vi "Read wires.vi"(8 "error in (no error)":errorcluster, 11 "BlockDiagram in":refnum<class "BlockDiagram.lvclass">) -> (0 "error out":errorcluster, 2 "wires":refnum<class "Wire.lvclass">[](array[class]), 3 "BlockDiagram out":refnum<class "BlockDiagram.lvclass">)   [LabVIEW 2023, in "TLC_Scripto.lvlib" / "BlockDiagram.lvclass"]
uses:
  BlockDiagram.lvclass
  Wire/Wire.lvclass
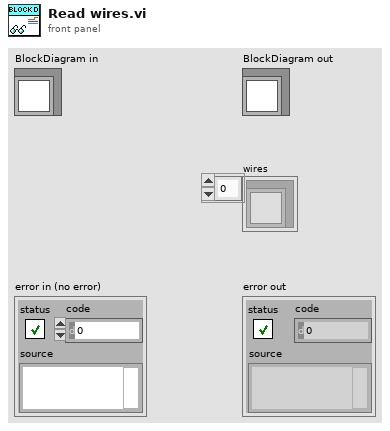
[diagram p1: front panel]
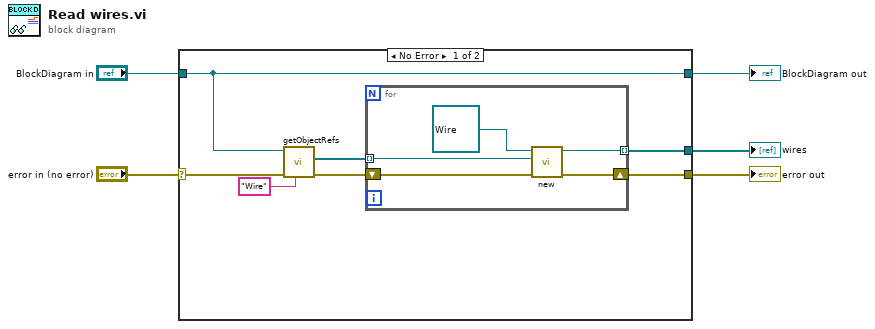
[diagram p0: block diagram]
diagram:
  n1 = case shown="No Error" "error in (no error)" {
    selector: "error in (no error)" -> [w10 w19]
    tunnel: [w7 w19] -> w4
    tunnel: [w12 w18] -> w2
    tunnel: "BlockDiagram in" -> [w12 w18]
    tunnel: [w6 _] -> w1
    frame No Error {
      n2 = call "getObjectRefs.vi"("type(ClassName)"="Wire" ("Class Name"), "error in (no error)"=w10, "BlockDiagram in"=w12) -> ("error out"=w8:errorcluster, "refs"=w9:refnum<vi>[])  [unwired: 6 in, 1 out]
      n3 = for {
        tunnel: w9 -> [w16] mode=indexing
        shift-right: [w14] -> w7
        shift-left: w8 -> [w15]
        tunnel: [w13] -> w6 mode=indexing
        n4 = call-dynamic "new.vi"("Error In"=w15, "ref"=w16, "Generic In"=refnum<class "Wire.lvclass"> refnum ("TLC_Scripto.lvlib:Wire")) -> ("Error Out"=w14:errorcluster, "Generic Out"=w13:refnum<class "Wire.lvclass">)  [unwired: 7 in]
      }
    }
    frame Error {
    }
  }
  "error out" <- w4
  "BlockDiagram out" <- w2
  "wires" <- w1
